vi "Get Controls.vi"(10 "Pnl Refnum":refnum<vi>) -> ()   [LabVIEW 2021]
uses:
  control info.ctl
  <vilib>/Utility/traverseref.llb/TRef TravTarget.ctl
  <vilib>/Utility/traverseref.llb/VI Scripting - Traverse.lvlib
panel:
  in  "Cancel":bool
  in  "Apply":bool
  in  "control info":T1[](array[typedef]) {"Boolean Type" items=["N/A", "FAB--icon--rounded", "outline--icon--rectangular", "outline--icon--rounded", "outline--text--rectangular", "outline--text--rounded", "nooutline--icon--rectangular", "nooutline--icon--rectangular--40x40", "nooutline--icon--rounded", "nooutline--text--rectangular", "nooutline--text--rounded", "tonal--icon--rectangular", "tonal--icon--rounded", "tonal--text--rectangular", "tonal--text--rounded", "filled--icon--rectangular", "filled--icon--rounded", "filled--text--rectangular", "filled--text--rounded"]; "UI Theme Level" items=["N/A", "Primary", "Secondary", "Tertiary", "Error", "Primary Fixed", "Secondary Fixed", "Tertiary Fixed", "Label Only", "No Change"]}
  out "error out":errorcluster
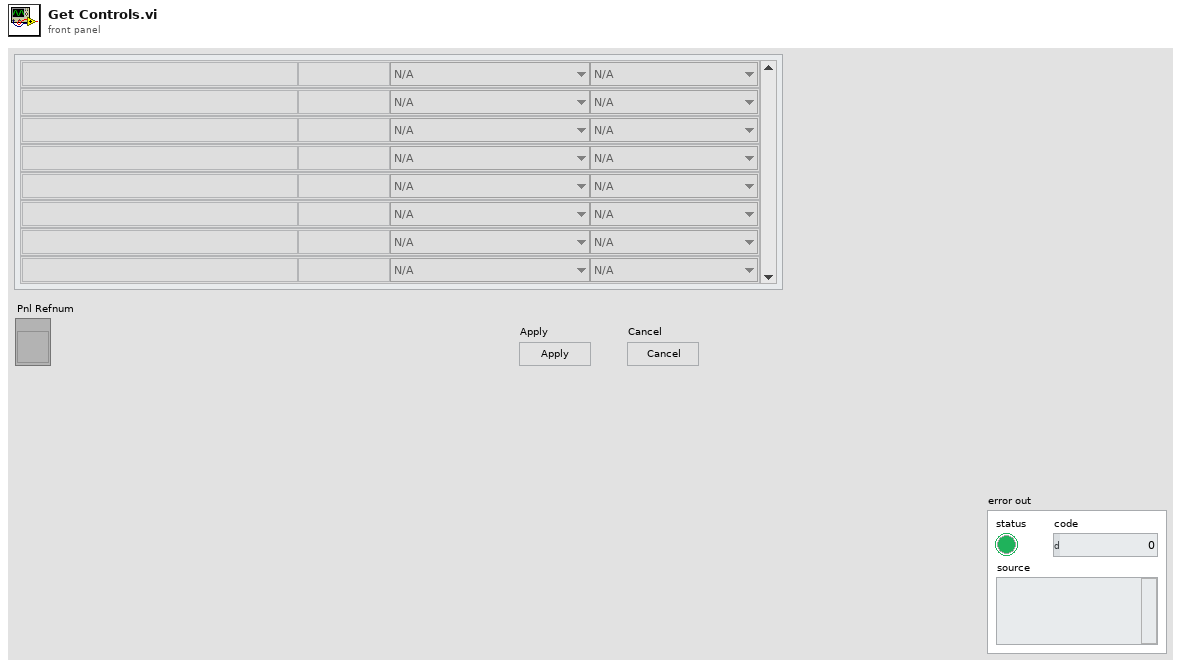
[diagram p1: front panel]
types:
  T1 = typedef "control info.ctl" = cluster{"label":string, "control type":string, "UI Theme Level":u16, "Boolean Type":u16}
  T2 = typedef "TRef TravTarget.ctl" = enum16{"FP", "BD", "Other"}
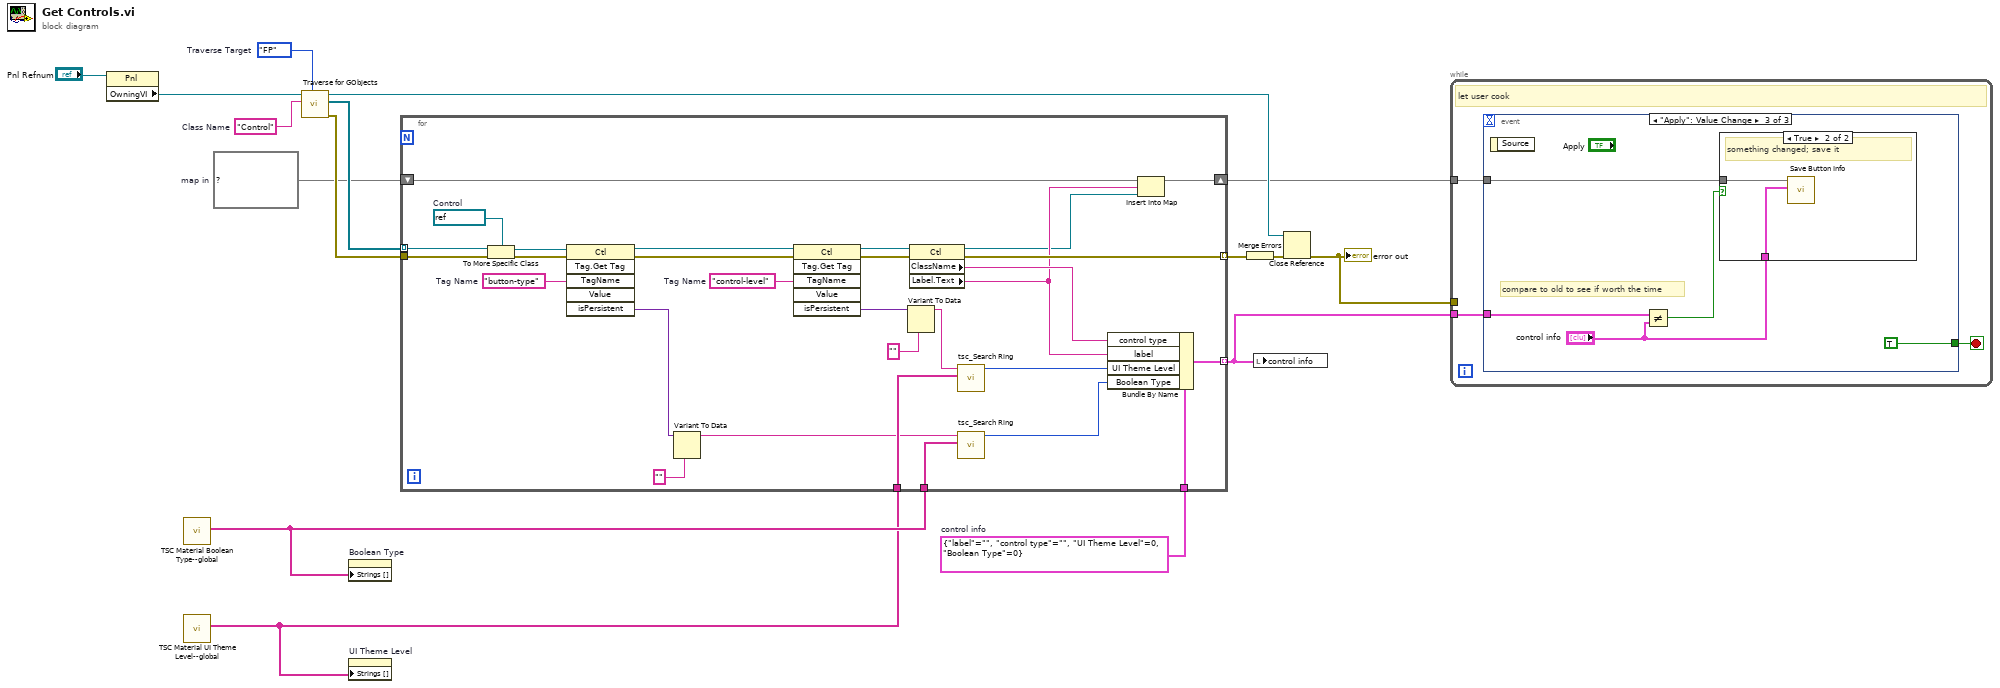
[diagram p0: block diagram]
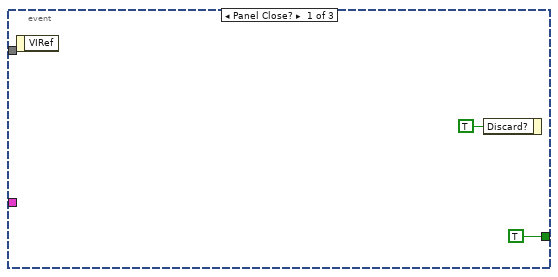
[diagram p2: hidden frame]
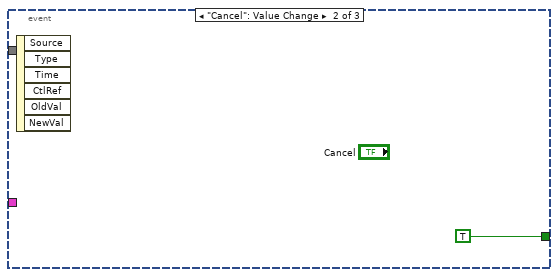
[diagram p3: hidden frame]
diagram:
  w2 = map{string, refnum<vi>} {}  # map in
  w9 = T1 {"label"="", "control type"="", "UI Theme Level"=0, "Boolean Type"=0}  # control info
  w15 = TRef_TravTarget."FP"  # Traverse Target
  w16 = "Control"  # Class Name
  n1 = property class="Pnl"(reference="Pnl Refnum") -> ("OwningVI"=w6:refnum<vi>)  [unwired: 1 in, 2 out]
  n2 = call "TSC Material Boolean Type--global.vi"() -> ("boolean types"=w8:string[])  [unwired: 11 in]
  n3 = call "TSC Material UI Theme Level--global.vi"() -> ("UI theme levels"=w7:string[])  [unwired: 11 in]
  n4 = call <vilib>:"Traverse for GObjects.vi"("Traverse Target"=w15, "Class Name"=w16, "VI Refnum"=w6) -> ("error out"=w13:errorcluster, "References"=w14:refnum<vi>[], "dup VI Refnum"=w5:refnum<vi>)  [unwired: 5 in, 1 out]
  n5 = property on="Boolean Type" class="Ring (strict)"("Strings []"=w8) -> ()  [unwired: 2 in, 2 out]
  n6 = property on="UI Theme Level" class="Ring (strict)"("Strings []"=w7) -> ()  [unwired: 2 in, 2 out]
  n7 = for {
    tunnel: w14 -> [w32] mode=indexing
    tunnel: w13 -> [w42]
    tunnel: [w35] -> w12 mode=indexing
    tunnel: w9 -> [w29]
    tunnel: w8 -> [w23]
    tunnel: [w27] -> w3 mode=indexing
    tunnel: w7 -> [w26]
    shift-right: [w19] -> w1
    shift-left: w2 -> [w20]
    w30 = refnum<vi> refnum  # Control
    w36 = "control-level"  # Tag Name
    w45 = "button-type"  # Tag Name
    n8 = To More Specific Class(target class=w30, reference=w32, error in=w42) -> (specific class reference=w31:refnum<vi>, error out=w33:errorcluster)
    n9 = invoke class="Ctl" method="Tag.Get Tag"(reference=w31, error in=w33, "TagName"=w45) -> (reference out=w39:refnum<vi>, error out=w41:errorcluster, "isPersistent"=w44:variant)  [unwired: 3 in, 3 out]
    n10 = Variant To Data(type="", Variant=w44) -> (data=w22:string)  [unwired: 1 in, 1 out]
    n11 = invoke class="Ctl" method="Tag.Get Tag"(reference=w39, error in=w41, "TagName"=w36) -> (reference out=w34:refnum<vi>, error out=w40:errorcluster, "isPersistent"=w37:variant)  [unwired: 3 in, 3 out]
    n12 = Variant To Data(type="", Variant=w37) -> (data=w25:string)  [unwired: 1 in, 1 out]
    n13 = property class="Ctl"(reference=w34, error in=w40) -> (reference out=w17:refnum<vi>, error out=w35:errorcluster, "ClassName"=w28:string, "Label.Text"=w18:string)
    n14 = call "tsc_Search Ring.vi"("Values"=w26, "Search Item"=w25) -> ("Index"=w24:u16)  [unwired: 9 in]
    n15 = call "tsc_Search Ring.vi"("Values"=w23, "Search Item"=w22) -> ("Index"=w21:u16)  [unwired: 9 in]
    n16 = Bundle By Name(cluster=w29, "control type"=w28, "label"=w18, "UI Theme Level"=w24, "Boolean Type"=w21) -> (w27:T1)
    n17 = Insert Into Map(map in=w20, key=w18, value=w17) -> (map out=w19:map{string, refnum<vi>})  [unwired: 2 out]
  }
  n18 = Merge Errors(w12) -> (w11:errorcluster)
  n19 = local write "control info"(w3) -> ()
  n20 = Close Reference(reference=w5, error in (no error)=w11) -> (error out=w4:errorcluster)
  "error out" <- w4
  n21 = while {
    tunnel: w4 -> [_]
    tunnel: w3 -> [w47]
    tunnel: w1 -> [w46]
    stop <- w48 stop-if-true
    # "let user cook"
    n22 = event shown="[2] \"Apply\": Value Change" {
      selector: _ -> [_ _ _]
      dyn-events: _ -> [_ _ _]
      timeout: _ -> [_ _ _]
      tunnel: [TRUE TRUE TRUE] -> w48
      tunnel: w47 -> [_ _ w55]
      tunnel: w46 -> [_ _ w54]
      event Panel Close? {
        n23 = event-data() -> ()  [unwired: 1 in, 1 out]
        n24 = event-data("Discard?"=TRUE) -> ()  [unwired: 1 in, 1 out]
      }
      event "Cancel": Value Change {
        n25 = event-data() -> ()  [unwired: 1 in, 6 out]
      }
      event "Apply": Value Change {
        # "compare to old to see if worth the time"
        n26 = event-data() -> ()  [unwired: 1 in, 1 out]
        n27 = Not Equal?(x=w55, y="control info") -> (x != y?=w52:bool)
        n28 = case shown="True" w52 {
          tunnel: w54 -> [_ w58]
          tunnel: "control info" -> [_ w57]
          frame False {
          }
          frame True {
            # "something changed; save it"
            n29 = call "Save Button Info.vi"("control info"=w57, "map in"=w58) -> ()  [unwired: 9 in, 1 out]
          }
        }
      }
    }
  }
